vi "ContainerOffset.vi"(9 "Lights Values":T1=[[{"Port"=1, "On Value"=255, "Off Value"=255}, {"Port"=2, "On Value"=0, "Off Value"=0}, {"Port"=3, "On Value"=0, "Off Value"=0}], [{"Port"=4, "On Value"=0, "Off Value"=0}, {"Port"=5, "On Value"=0, "Off Value"=0}, {"Port"=6, "On Value"=0, "Off Value"=0}], [{"Port"=7, "On Value"=0, "Off Value"=0}, {"Port"=8, "On Value"=0, "Off Value"=0}, {"Port"=9, "On Value"=0, "Off Value"=0}], [{"Port"=10, "On Value"=0, "Off Value"=0}, {"Port"=11, "On Value"=0, "Off Value"=0}, {"Port"=12, "On Value"=0, "Off Value"=0}], [{"Port"=13, "On Value"=0, "Off Value"=0}, {"Port"=14, "On Value"=0, "Off Value"=0}, {"Port"=15, "On Value"=0, "Off Value"=0}], [{"Port"=58, "On Value"=255, "Off Value"=0}, {"Port"=0, "On Value"=0, "Off Value"=0}, {"Port"=0, "On Value"=0, "Off Value"=0}], [{"Port"=49, "On Value"=255, "Off Value"=0}, {"Port"=0, "On Value"=0, "Off Value"=0}, {"Port"=0, "On Value"=0, "Off Value"=0}], [{"Port"=52, "On Value"=255, "Off Value"=0}, {"Port"=0, "On Value"=0, "Off Value"=0}, {"Port"=0, "On Value"=0, "Off Value"=0}], [{"Port"=55, "On Value"=255, "Off Value"=0}, {"Port"=0, "On Value"=0, "Off Value"=0}, {"Port"=0, "On Value"=0, "Off Value"=0}], [{"Port"=46, "On Value"=255, "Off Value"=0}, {"Port"=0, "On Value"=0, "Off Value"=0}, {"Port"=0, "On Value"=0, "Off Value"=0}], [{"Port"=61, "On Value"=0, "Off Value"=0}, {"Port"=0, "On Value"=0, "Off Value"=0}, {"Port"=0, "On Value"=0, "Off Value"=0}]], 10 "Buttons":bool[](array[boolean]), 11 "Presets":T2) -> ()   [LabVIEW 2014]
doc: "If the container/tote button is pressed, change value to 0 or offset and turn light on if the new value is the container offset"
uses:
  PresetValues.ctl
  LEDdriver/LEDPorts.ctl
  <vilib>/Rock Robotics/Network Tables/SD Read Number.vi
  <vilib>/Rock Robotics/Network Tables/SD Write Number.vi
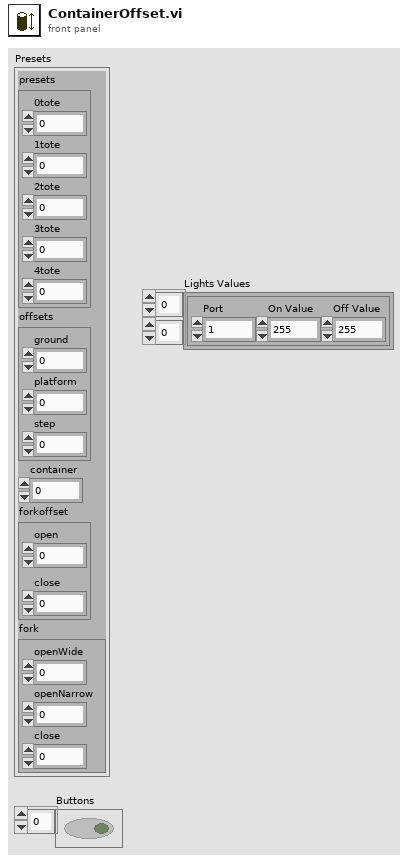
[diagram p1: front panel]
types:
  T1 = typedef "LEDPorts.ctl" = cluster{"Port":i16, "On Value":u8, "Off Value":u8}[][]
  T2 = typedef "PresetValues.ctl" = cluster{"presets":cluster{"0tote":dbl, "1tote":dbl, "2tote":dbl, "3tote":dbl, "4tote":dbl}, "offsets":cluster{"ground":dbl, "platform":dbl, "step":dbl}, "container":dbl, "forkoffset":cluster{"open":dbl, "close":dbl}, "fork":cluster{"openWide":dbl, "openNarrow":dbl, "close":dbl}}
  T3 = cluster{"Port":i16, "On Value":u8, "Off Value":u8}
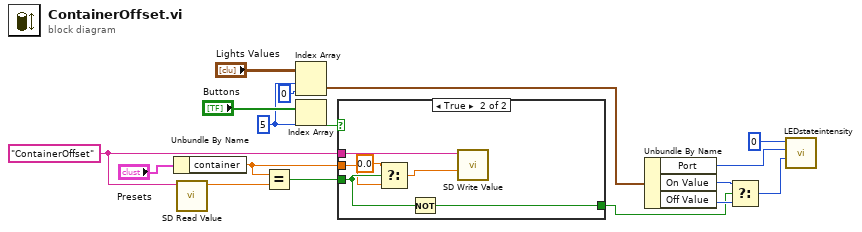
[diagram p0: block diagram]
diagram:
  w14 = "ContainerOffset" ("Name")
  w10 = 5 ("index")
  n1 = Unbundle By Name("Presets") -> ("container"=w13:dbl)
  n2 = call-poly <vilib>:"SD Read Value.vi"("Name"=w14) -> ("Numeric"=w12:dbl)  [unwired: 8 in, 2 out]
  n3 = Equal?(x=w13, y=w12) -> (x = y?=w2:bool)
  n4 = Index Array(array="Lights Values", index (row)=w10, index (col)=0 ("disabled index (col)")) -> (element=w8:T3)
  n5 = Index Array(array="Buttons", index=w10) -> (element=w17:bool)
  n6 = case shown="True" w17 {
    tunnel: w13 -> [_ w19]
    tunnel: w14 -> [_ w23]
    tunnel: w2 -> [w18 w22]
    tunnel: [w18 w21] -> w1
    frame False {
    }
    frame True {
      n7 = Select(t=0.0 ("f"), s=w22, f=w19) -> (s? t:f=w24:dbl)
      n8 = Not(x=w22) -> (.not. x?=w21:bool)
      n9 = call-poly <vilib>:"SD Write Value.vi"("Numeric"=w24, "Name"=w23) -> ()  [unwired: 8 in, 2 out]
    }
  }
  n10 = Unbundle By Name(w8) -> ("Port"=w6:i16, "On Value"=w5:u8, "Off Value"=w4:u8)
  n11 = Select(t=w5, s=w1, f=w4) -> (s? t:f=w3:u8)
  n12 = call "LEDstateintensity.vi"("intensity"=w3, "port"=w6, "Id"=i16 0) -> ()  [unwired: 6 in, 3 out]
